vi "Add tag to memory.vi"(8 "error in (no error)":errorcluster, 10 "Value":string, 11 "Data Type":T1) -> (0 "error out":errorcluster, 3 "Index":i32)   [LabVIEW 2010, in "Current Value Table.lvlib"]
uses:
  Current Value Table.lvlib
  Type Defs/Data Types.ctl
  Type Defs/Memory Commands.ctl
  DataTypes/Double_ASCII String To Data.vi
  DataTypes/Array of String_ASCII String To Data.vi
  DataTypes/Array of Boolean_ASCII String To Data.vi
  DataTypes/Array of Single_ASCII String To Data.vi
  DataTypes/Array of Double_ASCII String To Data.vi
  DataTypes/Array of I8_ASCII String To Data.vi
  DataTypes/Array of I16_ASCII String To Data.vi
  DataTypes/Array of I32_ASCII String To Data.vi
  DataTypes/Array of I64_ASCII String To Data.vi
  DataTypes/Array of U64_ASCII String To Data.vi
  DataTypes/Array of U32_ASCII String To Data.vi
  DataTypes/Array of U16_ASCII String To Data.vi
  DataTypes/Array of U8_ASCII String To Data.vi
  DataTypes/Boolean_ASCII String To Data.vi
  DataTypes/String_ASCII String To Data.vi
  DataTypes/U8_ASCII String To Data.vi
  DataTypes/U16_ASCII String To Data.vi
  DataTypes/U32_ASCII String To Data.vi
  DataTypes/U64_ASCII String To Data.vi
  DataTypes/I8_ASCII String To Data.vi
  DataTypes/I16_ASCII String To Data.vi
  DataTypes/I32_ASCII String To Data.vi
  DataTypes/I64_ASCII String To Data.vi
  DataTypes/Single_ASCII String To Data.vi
  Errors/Scanned Value Error.vi
  DataTypes/Double_Memory Block.vi
  DataTypes/Array of String_Memory Block.vi
  DataTypes/Array of Boolean_Memory Block.vi
  DataTypes/Array of Single_Memory Block.vi
  DataTypes/Array of Double_Memory Block.vi
  DataTypes/Array of I8_Memory Block.vi
  DataTypes/Array of I16_Memory Block.vi
  DataTypes/Array of I32_Memory Block.vi
  DataTypes/Array of I64_Memory Block.vi
  DataTypes/Array of U64_Memory Block.vi
  DataTypes/Array of U32_Memory Block.vi
  DataTypes/Array of U16_Memory Block.vi
  DataTypes/Array of U8_Memory Block.vi
  DataTypes/Boolean_Memory Block.vi
  DataTypes/String_Memory Block.vi
  DataTypes/U8_Memory Block.vi
  DataTypes/U16_Memory Block.vi
  DataTypes/U32_Memory Block.vi
  DataTypes/U64_Memory Block.vi
  DataTypes/I8_Memory Block.vi
  DataTypes/I16_Memory Block.vi
  DataTypes/I32_Memory Block.vi
  DataTypes/I64_Memory Block.vi
  DataTypes/Single_Memory Block.vi
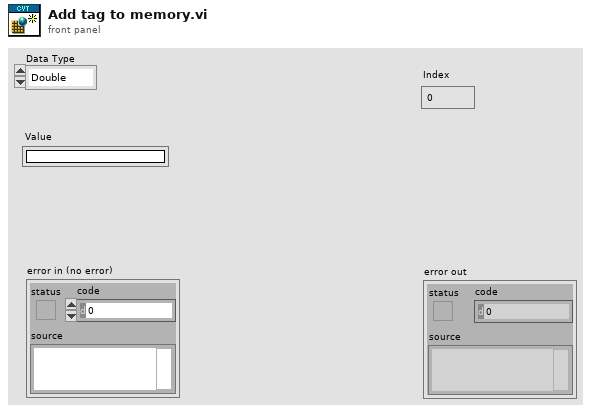
[diagram p1: front panel]
types:
  T1 = typedef "Current Value Table.lvlib/Data Types.ctl" = enum16{"Double", "Single", "I64", "I32", "I16", "I8", "U64", "U32", "U16", "U8", "String", "Boolean", "Array of U8", "Array of U16", "Array of U32", "Array of U64", "Array of I64", "Array of I32", "Array of I16", "Array of I8", "Array of Double", "Array of Single", "Array of Boolean", "Array of String"}
  T2 = typedef "Current Value Table.lvlib/Memory Commands.ctl" = enum16{"Init", "Add Data", "Read", "Read Group", "Read All", "Write", "Write Group", "Get Size"}
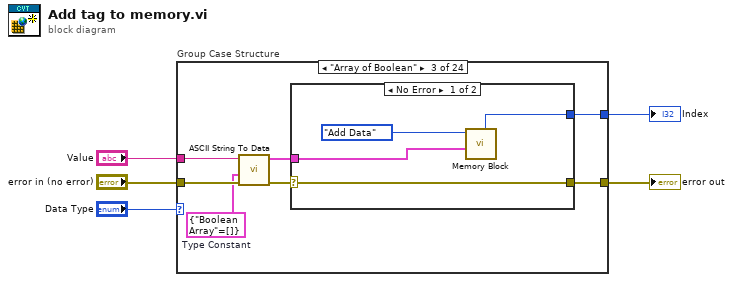
[diagram p0: block diagram]
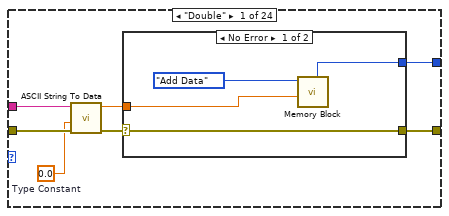
[diagram p2: hidden frame]
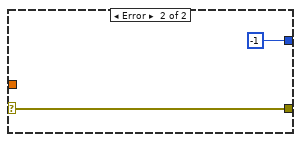
[diagram p3: hidden frame]
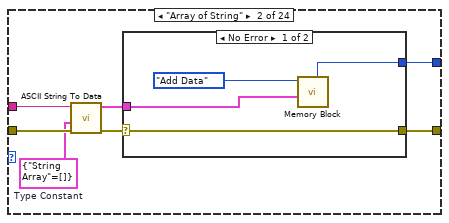
[diagram p4: hidden frame]
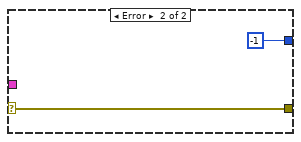
[diagram p5: hidden frame]
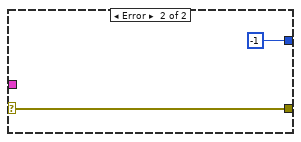
[diagram p6: hidden frame]
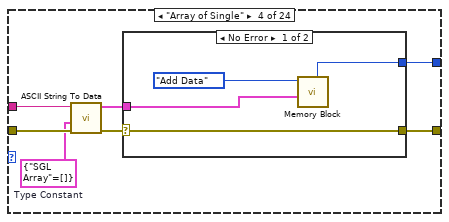
[diagram p7: hidden frame]
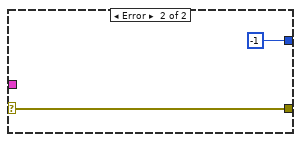
[diagram p8: hidden frame]
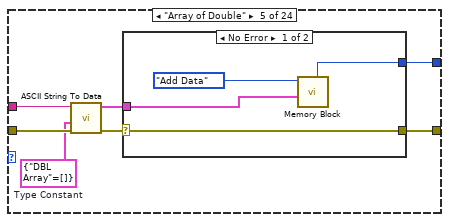
[diagram p9: hidden frame]
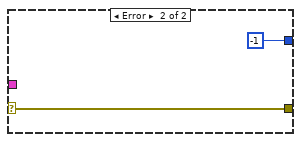
[diagram p10: hidden frame]
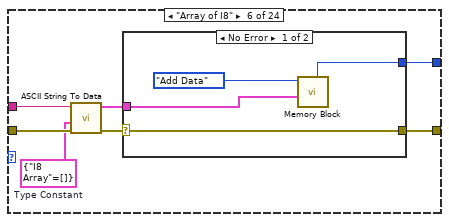
[diagram p11: hidden frame]
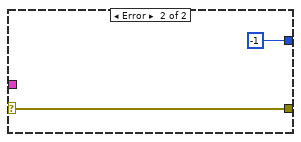
[diagram p12: hidden frame]
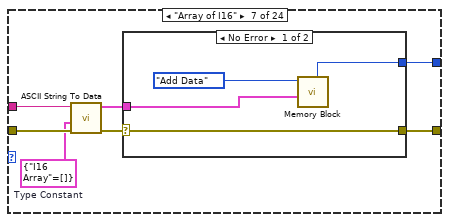
[diagram p13: hidden frame]
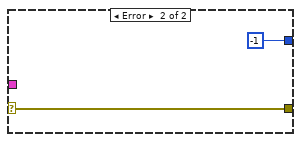
[diagram p14: hidden frame]
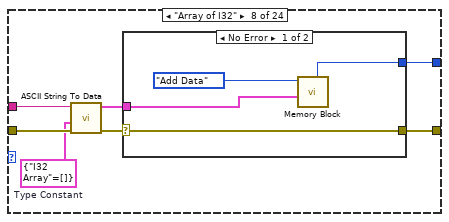
[diagram p15: hidden frame]
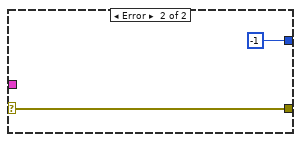
[diagram p16: hidden frame]
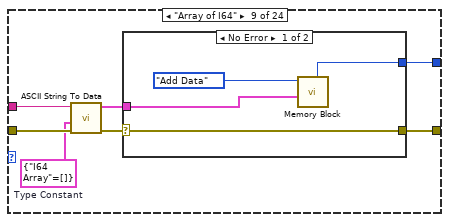
[diagram p17: hidden frame]
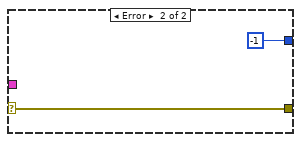
[diagram p18: hidden frame]
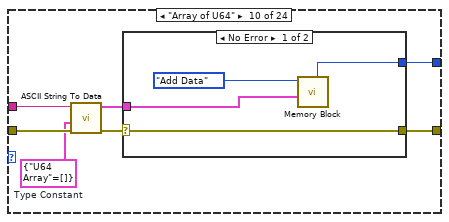
[diagram p19: hidden frame]
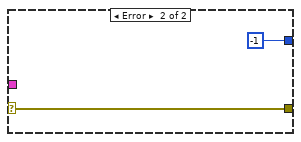
[diagram p20: hidden frame]
diagram:
  n1 = case "Group Case Structure" shown="\"Array of Boolean\"" "Data Type" {
    tunnel: "error in (no error)" -> [w12 w25 w38 w51 w64 w77 w90 w103 w116 w129 w142 w155 w168 w181 w194 w207 w220 w233 w246 w259 w272 w285 w298 w311]
    tunnel: "Value" -> [w11 w24 w37 w50 w63 w76 w89 w102 w115 w128 w141 w154 w167 w180 w193 w206 w219 w232 w245 w258 w271 w284 w297 w310]
    tunnel: [w9 w22 w35 w48 w61 w74 w87 w100 w113 w126 w139 w152 w165 w178 w191 w204 w217 w230 w243 w256 w269 w282 w295 w308] -> w5
    tunnel: [w8 w21 w34 w47 w60 w73 w86 w99 w112 w125 w138 w151 w164 w177 w190 w203 w216 w229 w242 w255 w268 w281 w294 w307] -> w4
    frame "Double" {
      w6 = 0.0  # Type Constant
      n2 = call-poly "ASCII String To Data.vi"("error in (no error)"=w12, "Default"=w6, "Value"=w11) -> ("error out"=w10:errorcluster, "Data"=w7:dbl)  [unwired: 7 in]
      n3 = case shown="No Error" w10 {
        selector: w10 -> [w14 w18]
        tunnel: w7 -> [w13 _]
        tunnel: [w15 -1 ("Array Size")] -> w9
        tunnel: [w14 w18] -> w8
        frame No Error {
          n4 = call-poly "Memory Block.vi"("Value"=w13, "Method"=Memory_Commands."Add Data") -> ("Array Size/Current Index"=w15:i32)  [unwired: 7 in, 2 out]
        }
        frame Error {
        }
      }
    }
    frame "Array of String" {
      w19 = cluster{"String Array":string[]} {"String Array"=[]}  # Type Constant
      n5 = call-poly "ASCII String To Data.vi"("error in (no error)"=w25, "Default"=w19, "Value"=w24) -> ("error out"=w23:errorcluster, "Data"=w20:cluster{"String Array":string[]})  [unwired: 7 in]
      n6 = case shown="No Error" w23 {
        selector: w23 -> [w27 w31]
        tunnel: w20 -> [w26 _]
        tunnel: [w28 -1 ("Array Size")] -> w22
        tunnel: [w27 w31] -> w21
        frame No Error {
          n7 = call-poly "Memory Block.vi"("Value"=w26, "Method"=Memory_Commands."Add Data") -> ("Array Size/Current Index"=w28:i32)  [unwired: 7 in, 2 out]
        }
        frame Error {
        }
      }
    }
    frame "Array of Boolean" {
      w32 = cluster{"Boolean Array":bool[]} {"Boolean Array"=[]}  # Type Constant
      n8 = call-poly "ASCII String To Data.vi"("error in (no error)"=w38, "Default"=w32, "Value"=w37) -> ("error out"=w36:errorcluster, "Data"=w33:cluster{"Boolean Array":bool[]})  [unwired: 7 in]
      n9 = case shown="No Error" w36 {
        selector: w36 -> [w40 w44]
        tunnel: w33 -> [w39 _]
        tunnel: [w41 -1 ("Array Size")] -> w35
        tunnel: [w40 w44] -> w34
        frame No Error {
          n10 = call-poly "Memory Block.vi"("Value"=w39, "Method"=Memory_Commands."Add Data") -> ("Array Size/Current Index"=w41:i32)  [unwired: 7 in, 2 out]
        }
        frame Error {
        }
      }
    }
    frame "Array of Single" {
      w45 = cluster{"SGL Array":sgl[]} {"SGL Array"=[]}  # Type Constant
      n11 = call-poly "ASCII String To Data.vi"("error in (no error)"=w51, "Default"=w45, "Value"=w50) -> ("error out"=w49:errorcluster, "Data"=w46:cluster{"SGL Array":sgl[]})  [unwired: 7 in]
      n12 = case shown="No Error" w49 {
        selector: w49 -> [w53 w57]
        tunnel: w46 -> [w52 _]
        tunnel: [w54 -1 ("Array Size")] -> w48
        tunnel: [w53 w57] -> w47
        frame No Error {
          n13 = call-poly "Memory Block.vi"("Value"=w52, "Method"=Memory_Commands."Add Data") -> ("Array Size/Current Index"=w54:i32)  [unwired: 7 in, 2 out]
        }
        frame Error {
        }
      }
    }
    frame "Array of Double" {
      w58 = cluster{"DBL Array":dbl[]} {"DBL Array"=[]}  # Type Constant
      n14 = call-poly "ASCII String To Data.vi"("error in (no error)"=w64, "Default"=w58, "Value"=w63) -> ("error out"=w62:errorcluster, "Data"=w59:cluster{"DBL Array":dbl[]})  [unwired: 7 in]
      n15 = case shown="No Error" w62 {
        selector: w62 -> [w66 w70]
        tunnel: w59 -> [w65 _]
        tunnel: [w67 -1 ("Array Size")] -> w61
        tunnel: [w66 w70] -> w60
        frame No Error {
          n16 = call-poly "Memory Block.vi"("Value"=w65, "Method"=Memory_Commands."Add Data") -> ("Array Size/Current Index"=w67:i32)  [unwired: 7 in, 2 out]
        }
        frame Error {
        }
      }
    }
    frame "Array of I8" {
      w71 = cluster{"I8 Array":i8[]} {"I8 Array"=[]}  # Type Constant
      n17 = call-poly "ASCII String To Data.vi"("error in (no error)"=w77, "Default"=w71, "Value"=w76) -> ("error out"=w75:errorcluster, "Data"=w72:cluster{"I8 Array":i8[]})  [unwired: 7 in]
      n18 = case shown="No Error" w75 {
        selector: w75 -> [w79 w83]
        tunnel: w72 -> [w78 _]
        tunnel: [w80 -1 ("Array Size")] -> w74
        tunnel: [w79 w83] -> w73
        frame No Error {
          n19 = call-poly "Memory Block.vi"("Value"=w78, "Method"=Memory_Commands."Add Data") -> ("Array Size/Current Index"=w80:i32)  [unwired: 7 in, 2 out]
        }
        frame Error {
        }
      }
    }
    frame "Array of I16" {
      w84 = cluster{"I16 Array":i16[]} {"I16 Array"=[]}  # Type Constant
      n20 = call-poly "ASCII String To Data.vi"("error in (no error)"=w90, "Default"=w84, "Value"=w89) -> ("error out"=w88:errorcluster, "Data"=w85:cluster{"I16 Array":i16[]})  [unwired: 7 in]
      n21 = case shown="No Error" w88 {
        selector: w88 -> [w92 w96]
        tunnel: w85 -> [w91 _]
        tunnel: [w93 -1 ("Array Size")] -> w87
        tunnel: [w92 w96] -> w86
        frame No Error {
          n22 = call-poly "Memory Block.vi"("Value"=w91, "Method"=Memory_Commands."Add Data") -> ("Array Size/Current Index"=w93:i32)  [unwired: 7 in, 2 out]
        }
        frame Error {
        }
      }
    }
    frame "Array of I32" {
      w97 = cluster{"I32 Array":i32[]} {"I32 Array"=[]}  # Type Constant
      n23 = call-poly "ASCII String To Data.vi"("error in (no error)"=w103, "Default"=w97, "Value"=w102) -> ("error out"=w101:errorcluster, "Data"=w98:cluster{"I32 Array":i32[]})  [unwired: 7 in]
      n24 = case shown="No Error" w101 {
        selector: w101 -> [w105 w109]
        tunnel: w98 -> [w104 _]
        tunnel: [w106 -1 ("Array Size")] -> w100
        tunnel: [w105 w109] -> w99
        frame No Error {
          n25 = call-poly "Memory Block.vi"("Value"=w104, "Method"=Memory_Commands."Add Data") -> ("Array Size/Current Index"=w106:i32)  [unwired: 7 in, 2 out]
        }
        frame Error {
        }
      }
    }
    frame "Array of I64" {
      w110 = cluster{"I64 Array":i64[]} {"I64 Array"=[]}  # Type Constant
      n26 = call-poly "ASCII String To Data.vi"("error in (no error)"=w116, "Default"=w110, "Value"=w115) -> ("error out"=w114:errorcluster, "Data"=w111:cluster{"I64 Array":i64[]})  [unwired: 7 in]
      n27 = case shown="No Error" w114 {
        selector: w114 -> [w118 w122]
        tunnel: w111 -> [w117 _]
        tunnel: [w119 -1 ("Array Size")] -> w113
        tunnel: [w118 w122] -> w112
        frame No Error {
          n28 = call-poly "Memory Block.vi"("Value"=w117, "Method"=Memory_Commands."Add Data") -> ("Array Size/Current Index"=w119:i32)  [unwired: 7 in, 2 out]
        }
        frame Error {
        }
      }
    }
    frame "Array of U64" {
      w123 = cluster{"U64 Array":u64[]} {"U64 Array"=[]}  # Type Constant
      n29 = call-poly "ASCII String To Data.vi"("error in (no error)"=w129, "Default"=w123, "Value"=w128) -> ("error out"=w127:errorcluster, "Data"=w124:cluster{"U64 Array":u64[]})  [unwired: 7 in]
      n30 = case shown="No Error" w127 {
        selector: w127 -> [w131 w135]
        tunnel: w124 -> [w130 _]
        tunnel: [w132 -1 ("Array Size")] -> w126
        tunnel: [w131 w135] -> w125
        frame No Error {
          n31 = call-poly "Memory Block.vi"("Value"=w130, "Method"=Memory_Commands."Add Data") -> ("Array Size/Current Index"=w132:i32)  [unwired: 7 in, 2 out]
        }
        frame Error {
        }
      }
    }
    frame "Array of U32" {
      w136 = cluster{"U32 Array":u32[]} {"U32 Array"=[]}  # Type Constant
      n32 = call-poly "ASCII String To Data.vi"("error in (no error)"=w142, "Default"=w136, "Value"=w141) -> ("error out"=w140:errorcluster, "Data"=w137:cluster{"U32 Array":u32[]})  [unwired: 7 in]
      n33 = case shown="No Error" w140 {
        selector: w140 -> [w144 w148]
        tunnel: w137 -> [w143 _]
        tunnel: [w145 -1 ("Array Size")] -> w139
        tunnel: [w144 w148] -> w138
        frame No Error {
          n34 = call-poly "Memory Block.vi"("Value"=w143, "Method"=Memory_Commands."Add Data") -> ("Array Size/Current Index"=w145:i32)  [unwired: 7 in, 2 out]
        }
        frame Error {
        }
      }
    }
    frame "Array of U16" {
      w149 = cluster{"U16 Array":u16[]} {"U16 Array"=[]}  # Type Constant
      n35 = call-poly "ASCII String To Data.vi"("error in (no error)"=w155, "Default"=w149, "Value"=w154) -> ("error out"=w153:errorcluster, "Data"=w150:cluster{"U16 Array":u16[]})  [unwired: 7 in]
      n36 = case shown="No Error" w153 {
        selector: w153 -> [w157 w161]
        tunnel: w150 -> [w156 _]
        tunnel: [w158 -1 ("Array Size")] -> w152
        tunnel: [w157 w161] -> w151
        frame No Error {
          n37 = call-poly "Memory Block.vi"("Value"=w156, "Method"=Memory_Commands."Add Data") -> ("Array Size/Current Index"=w158:i32)  [unwired: 7 in, 2 out]
        }
        frame Error {
        }
      }
    }
    frame "Array of U8" {
      w162 = cluster{"U8 Array":u8[]} {"U8 Array"=[]}  # Type Constant
      n38 = call-poly "ASCII String To Data.vi"("error in (no error)"=w168, "Default"=w162, "Value"=w167) -> ("error out"=w166:errorcluster, "Data"=w163:cluster{"U8 Array":u8[]})  [unwired: 7 in]
      n39 = case shown="No Error" w166 {
        selector: w166 -> [w170 w174]
        tunnel: w163 -> [w169 _]
        tunnel: [w171 -1 ("Array Size")] -> w165
        tunnel: [w170 w174] -> w164
        frame No Error {
          n40 = call-poly "Memory Block.vi"("Value"=w169, "Method"=Memory_Commands."Add Data") -> ("Array Size/Current Index"=w171:i32)  [unwired: 7 in, 2 out]
        }
        frame Error {
        }
      }
    }
    frame "Boolean" {
      w175 = FALSE  # bool
      n41 = call-poly "ASCII String To Data.vi"("error in (no error)"=w181, "Default"=w175, "Value"=w180) -> ("error out"=w179:errorcluster, "Data"=w176:bool)  [unwired: 7 in]
      n42 = case shown="No Error" w179 {
        selector: w179 -> [w183 w187]
        tunnel: w176 -> [w182 _]
        tunnel: [w184 -1 ("Array Size")] -> w178
        tunnel: [w183 w187] -> w177
        frame No Error {
          n43 = call-poly "Memory Block.vi"("Value"=w182, "Method"=Memory_Commands."Add Data") -> ("Array Size/Current Index"=w184:i32)  [unwired: 7 in, 2 out]
        }
        frame Error {
        }
      }
    }
    frame "String" {
      w188 = ""  # Type Constant
      n44 = call-poly "ASCII String To Data.vi"("error in (no error)"=w194, "Default"=w188, "Value"=w193) -> ("error out"=w192:errorcluster, "Data"=w189:string)  [unwired: 7 in]
      n45 = case shown="No Error" w192 {
        selector: w192 -> [w196 w200]
        tunnel: w189 -> [w195 _]
        tunnel: [w197 -1 ("Array Size")] -> w191
        tunnel: [w196 w200] -> w190
        frame No Error {
          n46 = call-poly "Memory Block.vi"("Value"=w195, "Method"=Memory_Commands."Add Data") -> ("Array Size/Current Index"=w197:i32)  [unwired: 7 in, 2 out]
        }
        frame Error {
        }
      }
    }
    frame "U8" {
      w201 = u8 0  # Type Constant
      n47 = call-poly "ASCII String To Data.vi"("error in (no error)"=w207, "Default"=w201, "Value"=w206) -> ("error out"=w205:errorcluster, "Data"=w202:u8)  [unwired: 7 in]
      n48 = case shown="No Error" w205 {
        selector: w205 -> [w209 w213]
        tunnel: w202 -> [w208 _]
        tunnel: [w210 -1 ("Array Size")] -> w204
        tunnel: [w209 w213] -> w203
        frame No Error {
          n49 = call-poly "Memory Block.vi"("Value"=w208, "Method"=Memory_Commands."Add Data") -> ("Array Size/Current Index"=w210:i32)  [unwired: 7 in, 2 out]
        }
        frame Error {
        }
      }
    }
    frame "U16" {
      w214 = u16 0  # Type Constant
      n50 = call-poly "ASCII String To Data.vi"("error in (no error)"=w220, "Default"=w214, "Value"=w219) -> ("error out"=w218:errorcluster, "Data"=w215:u16)  [unwired: 7 in]
      n51 = case shown="No Error" w218 {
        selector: w218 -> [w222 w226]
        tunnel: w215 -> [w221 _]
        tunnel: [w223 -1 ("Array Size")] -> w217
        tunnel: [w222 w226] -> w216
        frame No Error {
          n52 = call-poly "Memory Block.vi"("Value"=w221, "Method"=Memory_Commands."Add Data") -> ("Array Size/Current Index"=w223:i32)  [unwired: 7 in, 2 out]
        }
        frame Error {
        }
      }
    }
    frame "U32" {
      w227 = u32 0  # Type Constant
      n53 = call-poly "ASCII String To Data.vi"("error in (no error)"=w233, "Default"=w227, "Value"=w232) -> ("error out"=w231:errorcluster, "Data"=w228:u32)  [unwired: 7 in]
      n54 = case shown="No Error" w231 {
        selector: w231 -> [w235 w239]
        tunnel: w228 -> [w234 _]
        tunnel: [w236 -1 ("Array Size")] -> w230
        tunnel: [w235 w239] -> w229
        frame No Error {
          n55 = call-poly "Memory Block.vi"("Value"=w234, "Method"=Memory_Commands."Add Data") -> ("Array Size/Current Index"=w236:i32)  [unwired: 7 in, 2 out]
        }
        frame Error {
        }
      }
    }
    frame "U64" {
      w240 = u64 0  # Type Constant
      n56 = call-poly "ASCII String To Data.vi"("error in (no error)"=w246, "Default"=w240, "Value"=w245) -> ("error out"=w244:errorcluster, "Data"=w241:u64)  [unwired: 7 in]
      n57 = case shown="No Error" w244 {
        selector: w244 -> [w248 w252]
        tunnel: w241 -> [w247 _]
        tunnel: [w249 -1 ("Array Size")] -> w243
        tunnel: [w248 w252] -> w242
        frame No Error {
          n58 = call-poly "Memory Block.vi"("Value"=w247, "Method"=Memory_Commands."Add Data") -> ("Array Size/Current Index"=w249:i32)  [unwired: 7 in, 2 out]
        }
        frame Error {
        }
      }
    }
    frame "I8" {
      w253 = i8 0  # Type Constant
      n59 = call-poly "ASCII String To Data.vi"("error in (no error)"=w259, "Default"=w253, "Value"=w258) -> ("error out"=w257:errorcluster, "Data"=w254:i8)  [unwired: 7 in]
      n60 = case shown="No Error" w257 {
        selector: w257 -> [w261 w265]
        tunnel: w254 -> [w260 _]
        tunnel: [w262 -1 ("Array Size")] -> w256
        tunnel: [w261 w265] -> w255
        frame No Error {
          n61 = call-poly "Memory Block.vi"("Value"=w260, "Method"=Memory_Commands."Add Data") -> ("Array Size/Current Index"=w262:i32)  [unwired: 7 in, 2 out]
        }
        frame Error {
        }
      }
    }
    frame "I16" {
      w266 = i16 0  # Type Constant
      n62 = call-poly "ASCII String To Data.vi"("error in (no error)"=w272, "Default"=w266, "Value"=w271) -> ("error out"=w270:errorcluster, "Data"=w267:i16)  [unwired: 7 in]
      n63 = case shown="No Error" w270 {
        selector: w270 -> [w274 w278]
        tunnel: w267 -> [w273 _]
        tunnel: [w275 -1 ("Array Size")] -> w269
        tunnel: [w274 w278] -> w268
        frame No Error {
          n64 = call-poly "Memory Block.vi"("Value"=w273, "Method"=Memory_Commands."Add Data") -> ("Array Size/Current Index"=w275:i32)  [unwired: 7 in, 2 out]
        }
        frame Error {
        }
      }
    }
    frame "I32" {
      w279 = 0  # Type Constant
      n65 = call-poly "ASCII String To Data.vi"("error in (no error)"=w285, "Default"=w279, "Value"=w284) -> ("error out"=w283:errorcluster, "Data"=w280:i32)  [unwired: 7 in]
      n66 = case shown="No Error" w283 {
        selector: w283 -> [w287 w291]
        tunnel: w280 -> [w286 _]
        tunnel: [w288 -1 ("Array Size")] -> w282
        tunnel: [w287 w291] -> w281
        frame No Error {
          n67 = call-poly "Memory Block.vi"("Value"=w286, "Method"=Memory_Commands."Add Data") -> ("Array Size/Current Index"=w288:i32)  [unwired: 7 in, 2 out]
        }
        frame Error {
        }
      }
    }
    frame "I64" {
      w292 = i64 0  # Type Constant
      n68 = call-poly "ASCII String To Data.vi"("error in (no error)"=w298, "Default"=w292, "Value"=w297) -> ("error out"=w296:errorcluster, "Data"=w293:i64)  [unwired: 7 in]
      n69 = case shown="No Error" w296 {
        selector: w296 -> [w300 w304]
        tunnel: w293 -> [w299 _]
        tunnel: [w301 -1 ("Array Size")] -> w295
        tunnel: [w300 w304] -> w294
        frame No Error {
          n70 = call-poly "Memory Block.vi"("Value"=w299, "Method"=Memory_Commands."Add Data") -> ("Array Size/Current Index"=w301:i32)  [unwired: 7 in, 2 out]
        }
        frame Error {
        }
      }
    }
    frame "Single" {
      w305 = sgl 0.0  # Type Constant
      n71 = call-poly "ASCII String To Data.vi"("error in (no error)"=w311, "Default"=w305, "Value"=w310) -> ("error out"=w309:errorcluster, "Data"=w306:sgl)  [unwired: 7 in]
      n72 = case shown="No Error" w309 {
        selector: w309 -> [w313 w317]
        tunnel: w306 -> [w312 _]
        tunnel: [w314 -1 ("Array Size")] -> w308
        tunnel: [w313 w317] -> w307
        frame No Error {
          n73 = call-poly "Memory Block.vi"("Value"=w312, "Method"=Memory_Commands."Add Data") -> ("Array Size/Current Index"=w314:i32)  [unwired: 7 in, 2 out]
        }
        frame Error {
        }
      }
    }
  }
  "error out" <- w4
  "Index" <- w5
